vi "setChannelArray.vi"(8 "error in (no error)":errorcluster, 10 "ChannelArray":refnum<class "ChannelArray.lvclass">, 11 "StaticOutputEditor.lvclass in":refnum<class "StaticOutputEditor.lvclass">) -> (0 "error out":errorcluster, 3 "StaticOutputEditor.lvclass out":refnum<class "StaticOutputEditor.lvclass">)   [LabVIEW 2009, in "Views.lvlib" / "ScriptEditor.lvlib" / "StaticOutputEditor.lvclass"]
uses:
  StaticOutputEditor.lvclass
  Tools/DatabaseHelpers/Database Objects/ChannelArray/ChannelArray.lvclass
  StaticOutputEditor.lvclass/StaticOutputEditor.ctl
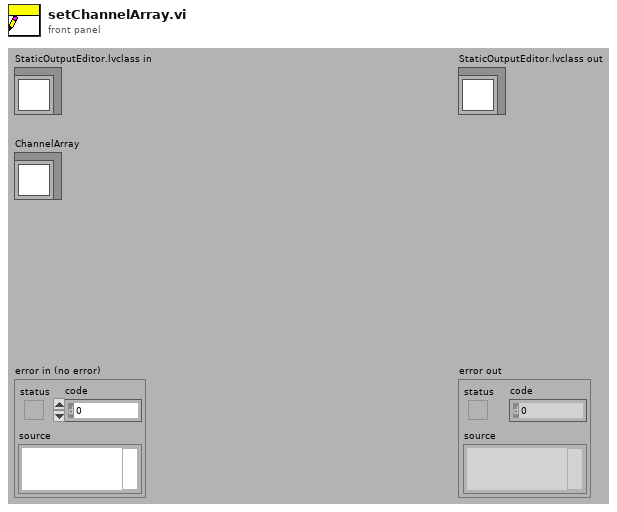
[diagram p1: front panel]
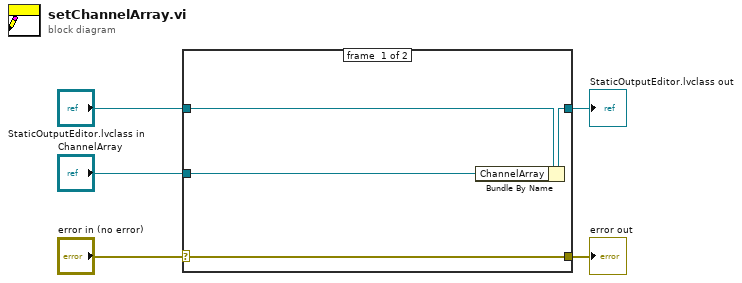
[diagram p0: block diagram]
diagram:
  n1 = case shown="No Error" "error in (no error)" {
    selector: "error in (no error)" -> [w9 w10]
    tunnel: [w9 w10] -> w4
    tunnel: [w7 w11] -> w2
    tunnel: "StaticOutputEditor.lvclass in" -> [w8 w11]
    tunnel: "ChannelArray" -> [w6 _]
    frame #0 {
      n2 = Bundle By Name(cluster=w8, "ChannelArray"=w6) -> (w7:refnum<class "StaticOutputEditor.lvclass">)
    }
    frame #1 {
    }
  }
  "error out" <- w4
  "StaticOutputEditor.lvclass out" <- w2
